vi "Reset UI.vi"(8 "error in (no error)":errorcluster, 11 "UserInterface in":refnum<class "UserInterface.lvclass">) -> (0 "error out":errorcluster, 3 "UserInterface out":refnum<class "UserInterface.lvclass">)   [LabVIEW 2021, in "UserInterface.lvlib" / "UserInterface.lvclass"]
uses:
  UserInterface.lvclass
  <vilib>/vision/Image Controls.llb/IMAQ Image.ctl
  UserInterface.lvclass/UserInterface.ctl
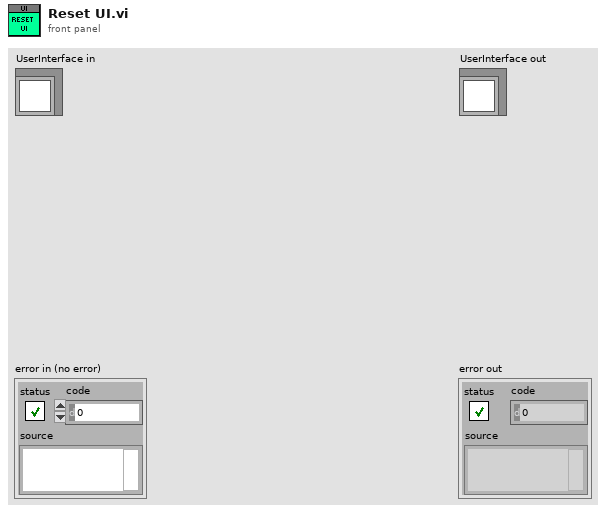
[diagram p1: front panel]
types:
  T1 = typedef "IMAQ Image.ctl" = refnum<image>
  T2 = cluster{"Image List":refnum<vi>, "ProgressBar":refnum<vi>, "Log":refnum<vi>, "Image Indicator":refnum<vi>}
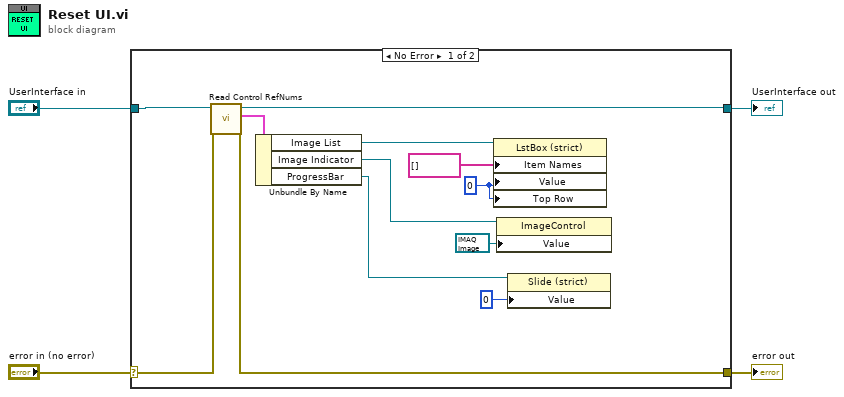
[diagram p0: block diagram]
diagram:
  n1 = case shown="No Error" "error in (no error)" {
    selector: "error in (no error)" -> [w16 w18]
    tunnel: [w15 w18] -> w3
    tunnel: [w9 w17] -> w1
    tunnel: "UserInterface in" -> [w14 w17]
    frame No Error {
      w10 = 0 ("Value")
      n2 = call "Read Control RefNums.vi"("error in (no error)"=w16, "UserInterface in"=w14) -> ("error out"=w15:errorcluster, "Control RefNums"=w13:T2, "UserInterface out"=w9:refnum<class "UserInterface.lvclass">)  [unwired: 7 in]
      n3 = Unbundle By Name(w13) -> ("Image List"=w12:refnum<vi>, "Image Indicator"=w8:refnum<vi>, "ProgressBar"=w6:refnum<vi>)
      n4 = property class="LstBox (strict)"(reference=w12, "Item Names"=string[] [], "Value"=w10, "Top Row"=w10) -> ()  [unwired: 1 in, 2 out]
      n5 = property class="ImageControl"(reference=w8, "Value"=T1 refnum ("Image")) -> ()  [unwired: 1 in, 2 out]
      n6 = property class="Slide (strict)"(reference=w6, "Value"=u32 0) -> ()  [unwired: 1 in, 2 out]
    }
    frame Error {
    }
  }
  "error out" <- w3
  "UserInterface out" <- w1
